vi "Public _Write Log.vi"(5 "Remark":string, 6 "Type":string, 7 "UserNo":string, 8 "error in (no error)":errorcluster caption="错误输入（无错误）", 9 "ErrMessage":string, 10 "Func":string, 11 "Traceability 引用句柄":refnum<k24>) -> (0 "error out":errorcluster caption="错误输出", 2 "Public_WriteLog":bool, 3 "Traceability 引用句柄输出":refnum<k24>)   [LabVIEW 2014, in "Traceability.lvlib"]
uses:
  D:/webservice/Traceability.dll
  Traceability.dll
  Traceability.lvlib
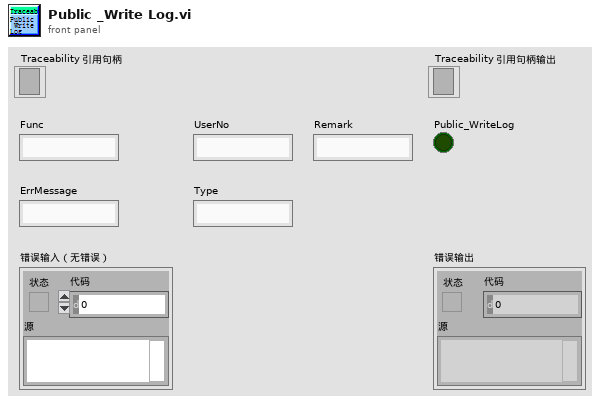
[diagram p1: front panel]
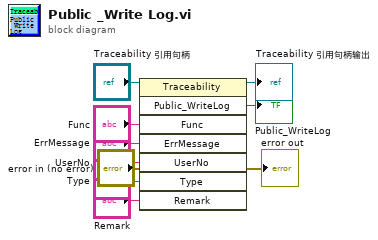
[diagram p0: block diagram]
diagram:
  n1 = invoke class="Traceability" method="Public_WriteLog"(reference="Traceability 引用句柄", error in="error in (no error)", "Func"="Func", "ErrMessage"="ErrMessage", "UserNo"="UserNo", "Type"="Type", "Remark"="Remark") -> (reference out=→"Traceability 引用句柄输出":refnum<k24>, error out=→"error out":errorcluster, "Public_WriteLog"=→"Public_WriteLog":bool)  [unwired: 1 in, 5 out]
